vi "VelocityRamp_r0 (SubVI).vi"(9 "Step Size":dbl=0.25 format="%#_13g", 10 "Current Velocity (RPS)":dbl, 11 "Input Velocity (RPS)":dbl) -> (3 "Output Velocity (RPS)":dbl)   [LabVIEW 2015]
panel:
  in  "Step Delay (ms)":u32=5
  in  "Threshold":dbl=0.25 format="%#_13g"
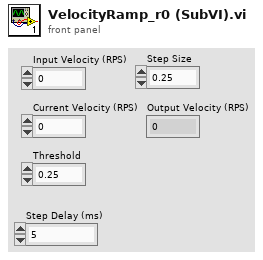
[diagram p1: front panel]
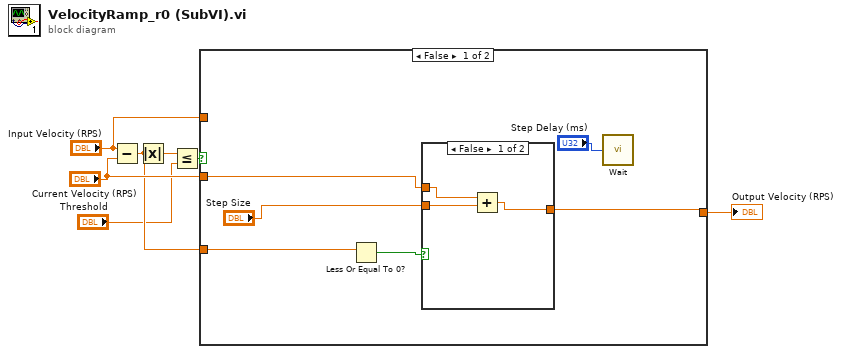
[diagram p0: block diagram]
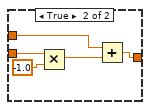
[diagram p2: hidden frame]
diagram:
  n1 = Subtract(x="Input Velocity (RPS)", y="Current Velocity (RPS)") -> (x-y=w5:dbl)
  n2 = Absolute Value(x=w5) -> (abs(x)=w4:dbl)
  n3 = Less Or Equal?(x=w4, y="Threshold") -> (x <= y?=w3:bool)
  n4 = case shown="False" w3 {
    tunnel: "Input Velocity (RPS)" -> [_ w22]
    tunnel: w5 -> [w13 _]
    tunnel: "Current Velocity (RPS)" -> [w12 _]
    tunnel: [w11 w22] -> w1
    frame False {
      n5 = Less Or Equal To 0?(x=w13) -> (x <= 0?=w10:bool)
      n6 = case shown="False" w10 {
        tunnel: "Step Size" -> [w15 w21]
        tunnel: w12 -> [w16 w19]
        tunnel: [w14 w17] -> w11
        frame False {
          n7 = Add(x=w16, y=w15) -> (x+y=w14:dbl)
        }
        frame True {
          n8 = Multiply(x=w21, y=-1.0) -> (x*y=w18:dbl)
          n9 = Add(x=w19, y=w18) -> (x+y=w17:dbl)
        }
      }
      n10 = call "Wait"("Count(mSec)"="Step Delay (ms)") -> ()  [unwired: 1 out]
    }
    frame True {
    }
  }
  "Output Velocity (RPS)" <- w1
